vi "Switch Checker.vi"(1 "Warning":bool, 2 "Correct Switch":bool) -> (0 "?":bool)   [LabVIEW 2024]
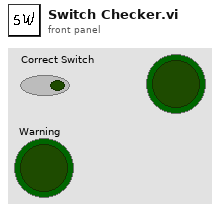
[diagram p1: front panel]
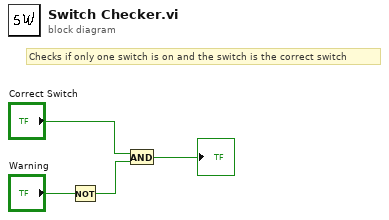
[diagram p0: block diagram]
diagram:
  # "Checks if only one switch is on and the switch is the correct switch"
  n1 = Not(x="Warning") -> (.not. x?=w4:bool)
  n2 = And(x="Correct Switch", y=w4) -> (x .and. y?=→"?":bool)
